vi "TP_Main.vi"() -> ()   [LabVIEW 2012]
panel:
  out "error out":errorcluster
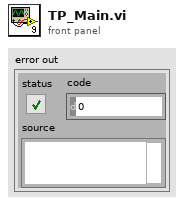
[diagram p1: front panel]
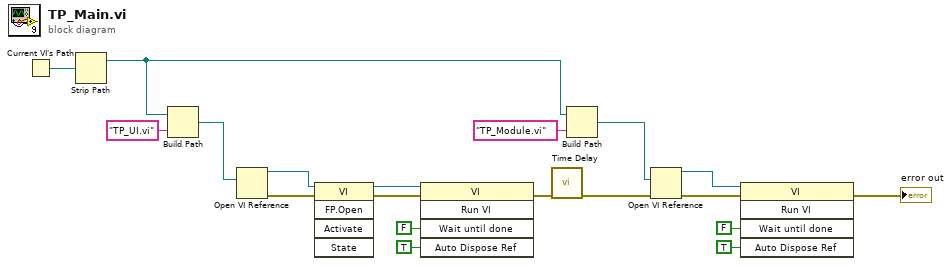
[diagram p0: block diagram]
diagram:
  n1 = Current VI's Path() -> (path=w7:path)
  n2 = Strip Path(path=w7) -> (stripped path=w3:path)  [unwired: 1 out]
  n3 = Build Path(base path=w3, name or relative path="TP_UI.vi") -> (appended path=w5:path)
  n4 = Open VI Reference(vi path=w5) -> (vi reference=w11:refnum<vi>, error out=w10:errorcluster)  [unwired: 5 in]
  n5 = invoke class="VI" method="FP.Open"(reference=w11, error in=w10) -> (reference out=w12:refnum<vi>, error out=w13:errorcluster)  [unwired: 3 in, 3 out]
  n6 = invoke class="VI" method="Run VI"(reference=w12, error in=w13, "Wait until done"=FALSE ("Wait Until Done"), "Auto Dispose Ref"=TRUE ("Auto Dispose Reference")) -> (error out=w14:errorcluster)  [unwired: 1 in, 4 out]
  n7 = call "Time Delay"("error in (no error)"=w14) -> ("error out"=w9:errorcluster)  [unwired: 10 in]
  n8 = Build Path(base path=w3, name or relative path="TP_Module.vi") -> (appended path=w2:path)
  n9 = Open VI Reference(vi path=w2, error in (no error)=w9) -> (vi reference=w19:refnum<vi>, error out=w8:errorcluster)  [unwired: 4 in]
  n10 = invoke class="VI" method="Run VI"(reference=w19, error in=w8, "Wait until done"=FALSE ("Wait Until Done"), "Auto Dispose Ref"=TRUE ("Auto Dispose Reference")) -> (error out=→"error out":errorcluster)  [unwired: 1 in, 4 out]
